vi "getDataFilePython.vi"(8 "error in (no error)":errorcluster, 11 "reference in":refnum<class "excelFile.lvclass">) -> (0 "error out":errorcluster, 3 "reference out":refnum<class "excelFile.lvclass">)   [LabVIEW 2015, in "excelFile.lvclass"]
uses:
  excelFile.lvclass
  python_class/python.lvclass
panel:
  out "Array":string[][][](array[string])
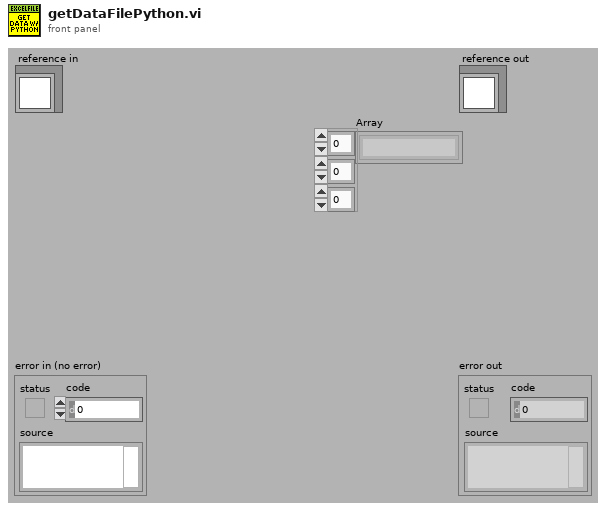
[diagram p1: front panel]
types:
  T1 = typedef "excelFile.lvclass/ObjectAttributesRef.ctl" = refnum<data-value>
  T2 = typedef "excelFile.lvclass/ObjectAttributes.ctl" = cluster{"MyAttribute":dbl, "path":string, "Refnum Excel":cluster{"Excel._Application":refnum<k7>, "Workbooks":refnum<k7>, "Open":refnum<k7>}, "data":string[][][], "save":bool, "fileType":T3, "rowsColor":u32[], "python_ref":refnum<class "python.lvclass">, "items_rows":i32[], "excel_range":i32[][]}
  T3 = typedef "excelFile.lvclass/fileType.ctl" = enum16{"devices", "items", "partsTracking", "TSR"}
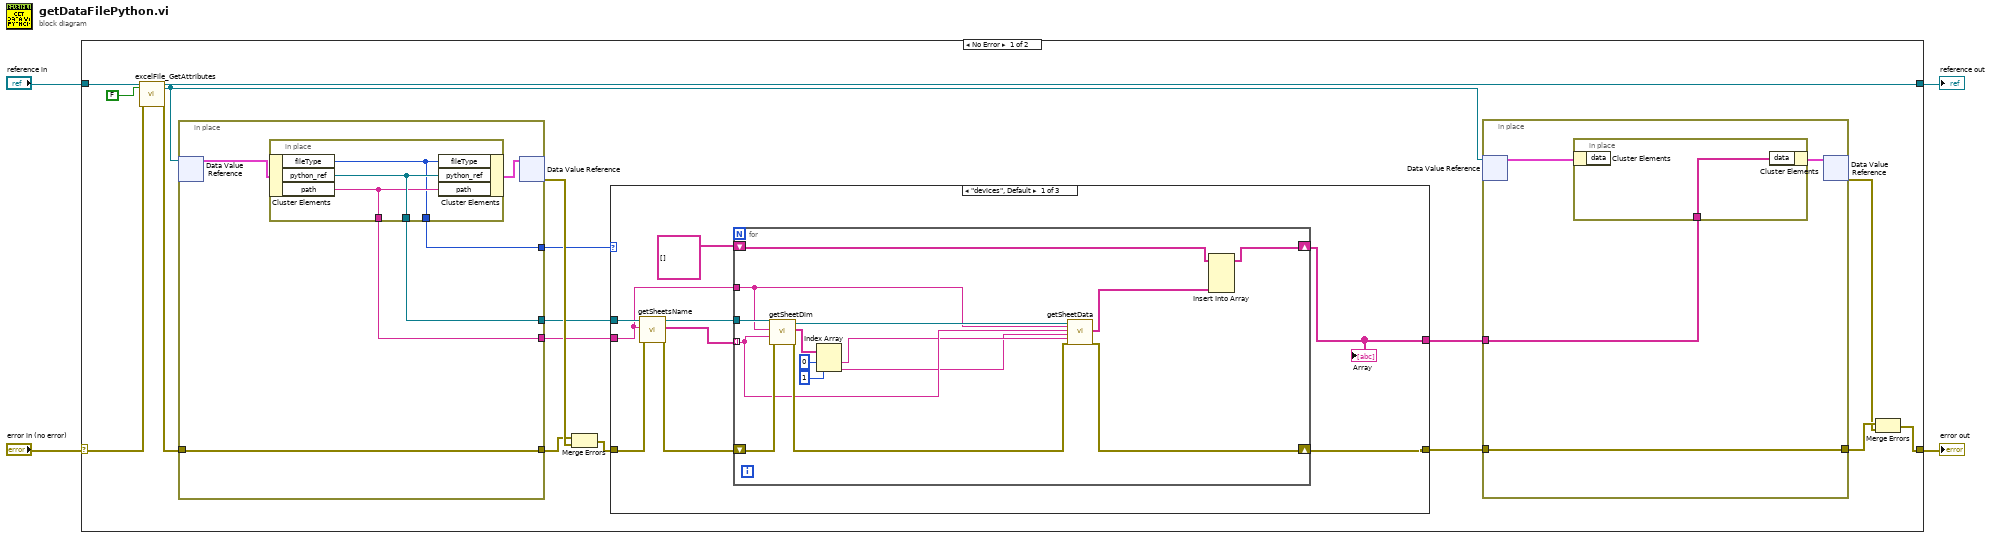
[diagram p0: block diagram]
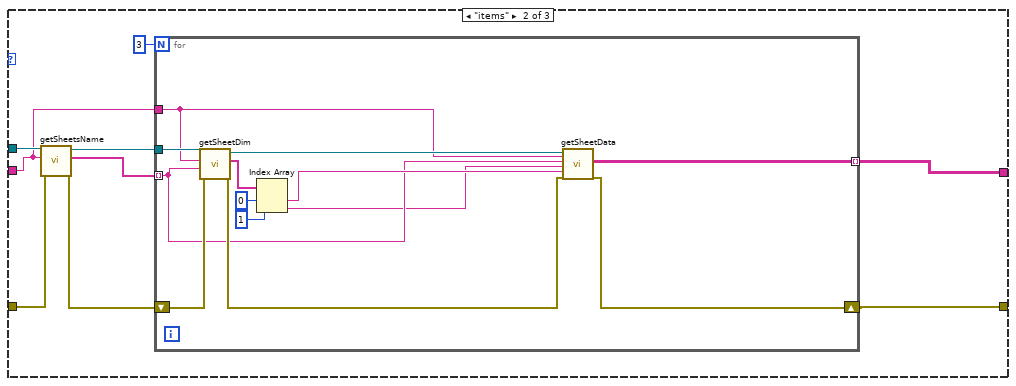
[diagram p2: hidden frame]
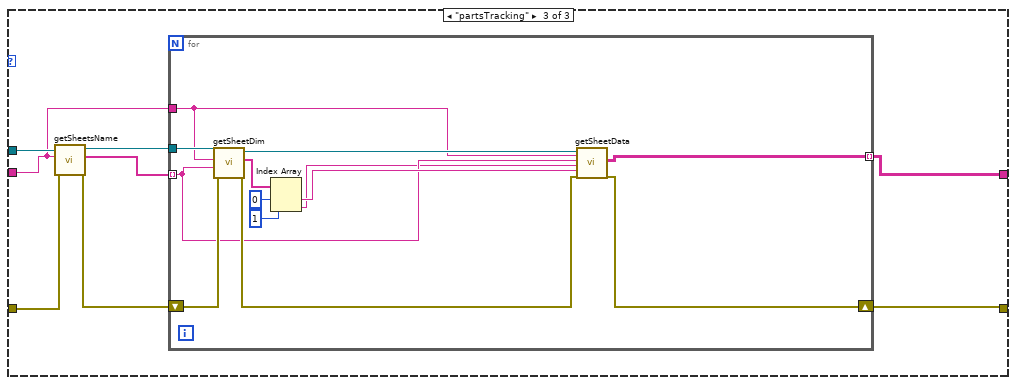
[diagram p3: hidden frame]
diagram:
  n1 = case shown="No Error" "error in (no error)" {
    selector: "error in (no error)" -> [w17 w104]
    tunnel: [w9 w104] -> w3
    tunnel: [w14 w103] -> w1
    tunnel: "reference in" -> [w19 w103]
    frame No Error {
      n2 = call "excelFile_GetAttributes.vi"("reference in"=w19, "return data? (T)"=FALSE, "error in (no error)"=w17) -> ("reference out"=w14:refnum<class "excelFile.lvclass">, "attributes ref"=w12:T1, "error out"=w16:errorcluster)  [unwired: 13 in, 1 out]
      n3 = in-place {
        in-place-border: w16 -> [w97]
        in-place-border: [w97] -> w20
        in-place-border: [w96] -> w7
        in-place-border: [w95] -> w6
        in-place-border: [w94] -> w8
        n4 = in-place-dvr #1(w12) -> (w98:T2)  [unwired: 1 out]
        n5 = in-place {
          in-place-border: [w102] -> w96
          in-place-border: [w101] -> w95
          in-place-border: [w100] -> w94
          n6 = in-place-cluster #2(w98) -> ("fileType"=w100:T3, "python_ref"=w102:refnum<class "python.lvclass">, "path"=w101:string)
          n7 = in-place-cluster #2("fileType"=w100, "python_ref"=w102, "path"=w101) -> (w99:T2)
        }
        n8 = in-place-dvr #1(w99) -> (w21:errorcluster)  [unwired: 1 out]
      }
      n9 = Merge Errors(w20, w21) -> (w15:errorcluster)
      n10 = case shown="\"devices\", Default" w8 {
        tunnel: w15 -> [w34 w56 w77]
        tunnel: [w32 w52 w73] -> w13
        tunnel: [w27 w53 w74] -> w5
        tunnel: w7 -> [w35 w55 w76]
        tunnel: w6 -> [w29 w54 w75]
        frame "devices", Default {
          n11 = call "getSheetsName.vi"("error in (no error)"=w34, "filePath"=w29, "reference in"=w35) -> ("error out"=w33:errorcluster, "sheetsName"=w30:string[], "reference out"=w31:refnum<class "python.lvclass">)  [unwired: 6 in]
          n12 = for {
            shift-right: [w49] -> w32
            shift-left: w33 -> [w47]
            tunnel: w31 -> [w50]
            tunnel: w30 -> [w42] mode=indexing
            tunnel: w29 -> [w41]
            shift-right: [w38] -> w27
            shift-left: string[][][] [] -> [w39]
            n13 = call "getSheetDim.vi"("error in (no error)"=w47, "sheetName"=w42, "filePath"=w41, "reference in"=w50) -> ("error out"=w46:errorcluster, "sheetsDim(Row,Column)"=w45:string[], "reference out"=w48:refnum<class "python.lvclass">)  [unwired: 5 in]
            n14 = Index Array(array=w45, index #1=0 ("index"), index #2=1 ("index")) -> (element #1=w37:string, element #2=w36:string)
            n15 = call "getSheetData.vi"("reference in"=w48, "filePath"=w41, "sheetName"=w42, "column"=w36, "row"=w37, "error in (no error)"=w46) -> ("dataOut"=w40:string[][], "error out"=w49:errorcluster)  [unwired: 11 in, 1 out]
            n16 = Insert Into Array(array=w39, new element=w40) -> (w38:string[][][])  [unwired: 3 in]
          }
          "Array" <- w27
        }
        frame "items" {
          n17 = call "getSheetsName.vi"("error in (no error)"=w56, "filePath"=w54, "reference in"=w55) -> ("error out"=w59:errorcluster, "sheetsName"=w57:string[], "reference out"=w58:refnum<class "python.lvclass">)  [unwired: 6 in]
          n18 = for {
            N: 3 -> [_]
            shift-right: [w71] -> w52
            shift-left: w59 -> [w69]
            tunnel: w58 -> [w72]
            tunnel: w57 -> [w63] mode=indexing
            tunnel: w54 -> [w62]
            tunnel: [w60] -> w53 mode=indexing
            n19 = call "getSheetDim.vi"("error in (no error)"=w69, "sheetName"=w63, "filePath"=w62, "reference in"=w72) -> ("error out"=w68:errorcluster, "sheetsDim(Row,Column)"=w67:string[], "reference out"=w70:refnum<class "python.lvclass">)  [unwired: 5 in]
            n20 = Index Array(array=w67, index #1=0 ("index"), index #2=1 ("index")) -> (element #1=w64:string, element #2=w61:string)
            n21 = call "getSheetData.vi"("reference in"=w70, "filePath"=w62, "sheetName"=w63, "column"=w61, "row"=w64, "error in (no error)"=w68) -> ("dataOut"=w60:string[][], "error out"=w71:errorcluster)  [unwired: 11 in, 1 out]
          }
        }
        frame "partsTracking" {
          n22 = call "getSheetsName.vi"("error in (no error)"=w77, "filePath"=w75, "reference in"=w76) -> ("error out"=w80:errorcluster, "sheetsName"=w78:string[], "reference out"=w79:refnum<class "python.lvclass">)  [unwired: 6 in]
          n23 = for {
            shift-right: [w92] -> w73
            shift-left: w80 -> [w90]
            tunnel: w79 -> [w93]
            tunnel: w78 -> [w84] mode=indexing
            tunnel: w75 -> [w83]
            tunnel: [w82] -> w74 mode=indexing
            n24 = call "getSheetDim.vi"("error in (no error)"=w90, "sheetName"=w84, "filePath"=w83, "reference in"=w93) -> ("error out"=w89:errorcluster, "sheetsDim(Row,Column)"=w88:string[], "reference out"=w91:refnum<class "python.lvclass">)  [unwired: 5 in]
            n25 = Index Array(array=w88, index #1=0 ("index"), index #2=1 ("index")) -> (element #1=w85:string, element #2=w81:string)
            n26 = call "getSheetData.vi"("reference in"=w91, "filePath"=w83, "sheetName"=w84, "column"=w81, "row"=w85, "error in (no error)"=w89) -> ("dataOut"=w82:string[][], "error out"=w92:errorcluster)  [unwired: 11 in, 1 out]
          }
        }
      }
      n27 = in-place {
        in-place-border: w13 -> [w23]
        in-place-border: [w23] -> w11
        in-place-border: w5 -> [w22]
        n28 = in-place-dvr #3(w12) -> (w24:T2)  [unwired: 1 out]
        n29 = in-place {
          in-place-border: w22 -> [w26]
          n30 = in-place-cluster #4(w24) -> ()  [unwired: 1 out]
          n31 = in-place-cluster #4("data"=w26) -> (w25:T2)
        }
        n32 = in-place-dvr #3(w25) -> (w10:errorcluster)  [unwired: 1 out]
      }
      n33 = Merge Errors(w11, w10) -> (w9:errorcluster)
    }
    frame Error {
    }
  }
  "error out" <- w3
  "reference out" <- w1
